vi "CRC_CCITT.vi"(4 "error in (no error)":errorcluster, 6 "CRC-CCITT Type (Initialization value)":u16(ring)=65535 format="%04x" items=["CRC-16-CCITT (0x1D0F)"=7439, "CRC-16-CCITT (0xFFFF)"=65535, "CRC-16-CCITT (XModem)"=0], 7 "unsigned byte array":u8[](array[numeric]) format="%.0x") -> (0 "error out":errorcluster, 2 "CRC array":u8[](array[numeric]) format="%02x", 3 "CRC-CCITT":u16 format="%x")   [LabVIEW 2015, in "Error Correction.lvlib"]
uses:
  Error Correction.lvlib
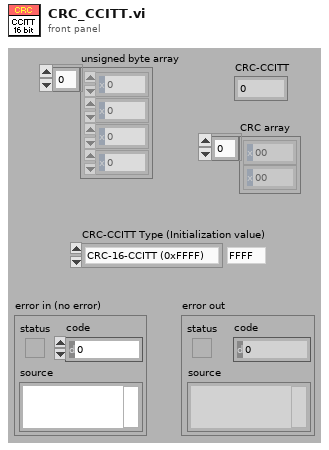
[diagram p1: front panel]
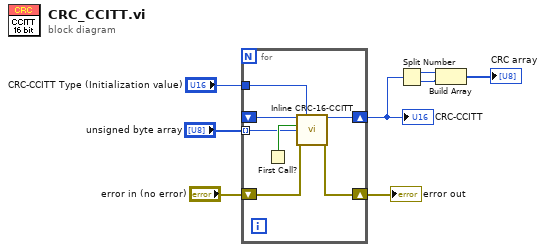
[diagram p0: block diagram]
diagram:
  n1 = for {
    shift-right: [w14] -> w7
    shift-left: _ -> [w15]
    tunnel: "unsigned byte array" -> [w12] mode=indexing
    tunnel: "CRC-CCITT Type (Initialization value)" -> [w11]
    shift-right: [w9] -> w1
    shift-left: "error in (no error)" -> [w10]
    n2 = First Call?() -> (First Call?: T/F=w13:bool)
    n3 = call "Inline CRC-16-CCITT.vi"("CRC In"=w15, "CRC-CCITT Type"=w11, "Reset"=w13, "Data"=w12, "error in (no error)"=w10) -> ("CRC"=w14:u16, "error out"=w9:errorcluster)  [unwired: 9 in]
  }
  "CRC-CCITT" <- w7
  "error out" <- w1
  n4 = Split Number(x=w7) -> (hi(x)=w6:u8, lo(x)=w5:u8)
  n5 = Build Array(w6, w5) -> (→"CRC array":u8[])
